vi "xyz-dh_express.vi"(0 "Image":dbl[][](array[numeric]), 1 "FFT":T2, 2 "Sizes":T1, 5 "R":dbl, 9 "Threshold type":u16(ring) items=["Top fraction", "Top value"], 11 "Threshold":dbl=2.0, 12 "FFT allocated?":bool=TRUE, 13 "mid_rng":dbl) -> (4 "XYZ":dbl[](array[numeric]), 6 "G":dbl[][](graph), 8 "Gx":dbl[][](graph), 10 "Gy":dbl[][](graph), 14 "dR":dbl[](array[numeric]), 15 "Filtered G":dbl[][](graph))   [LabVIEW 2015]
doc: "Single vi for calculating XYZ position of the particle.\n\nINPUT\nImage - input image\nR - radius of the window (should be >0.5)\nThreshold type, - type of threshold to apply:\n \"Top fraction\" - sets threshold as max_intensity/Threshold, e.g., for a Threshold=2 the threshold will be set to half the maximum pixel value \n \"Top value\" - sets the threshold to Threshold\nThreshold - threshold value\nFFT allocated? - must be set to true (default) if FFT and Sizes are connected. If set to False, FFT and Sizes inputs are ignored\nFFT, Sizes - Fourier transforms and sizes obtained from Local gradient preallocation\nPositive angle - angle in degrees that defines orientation of the image of the particle which corresponds to positive z-value\n\nOUTPUT\nXYZ - x,y position of the particle in pixels (for original image), z-value\nFiltered G - filtered local gradient magnitude image\nG,Gx,Gy - magnitude, horizontal and vertical local gradients correspondingly.\ndR - distance from the center to each line (1D vector)\n\nAuthor: Anatolii Kashchuk"
panel:
  in  "Weights type":u16(ring)=1 items=["None", "G", "G^2"]
  # "Author: Anatolii Kashchuk"
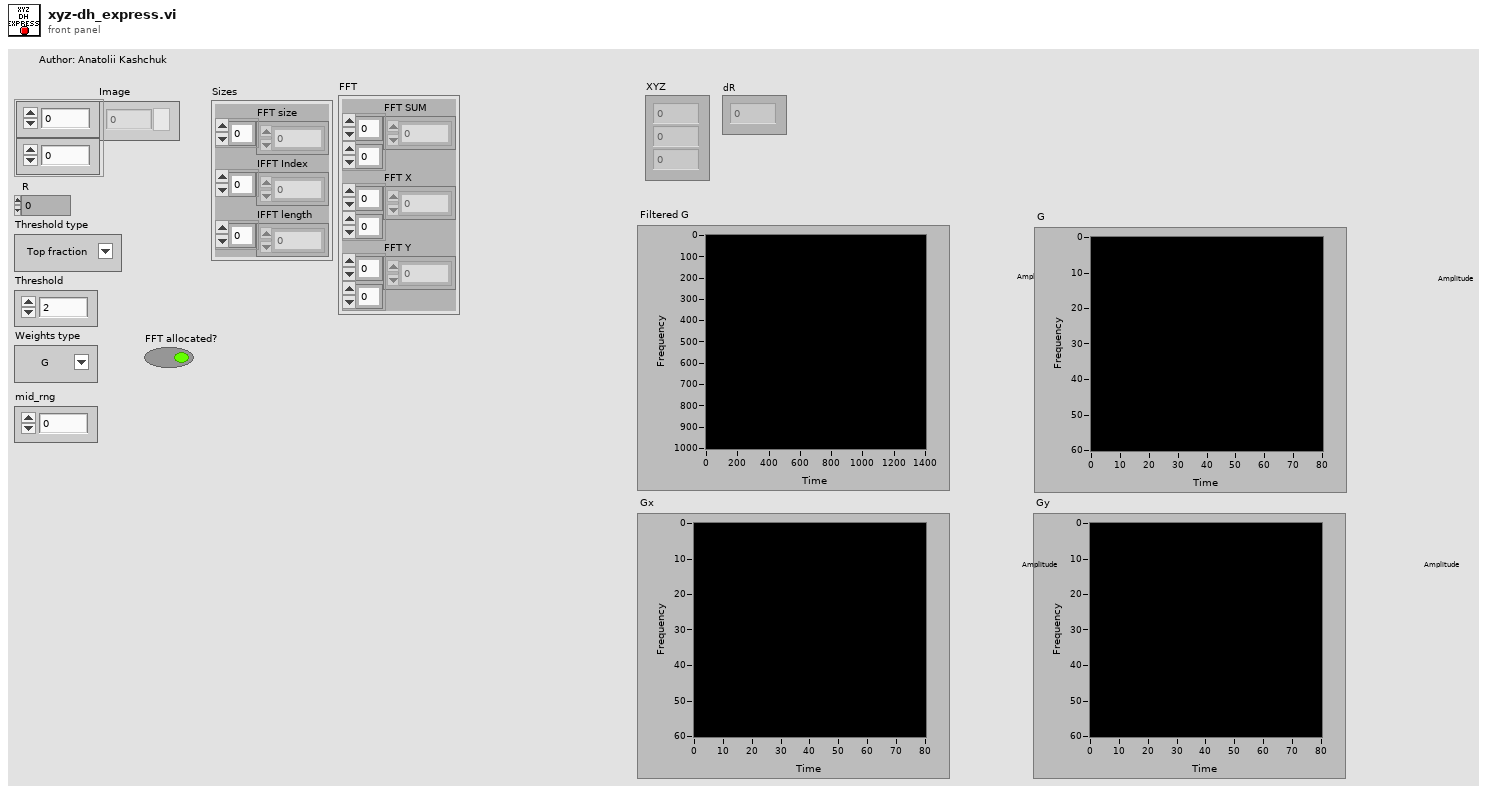
[diagram p1: front panel]
types:
  T1 = cluster{"FFT size":u32[], "IFFT Index":i32[], "IFFT length":u32[]}
  T2 = cluster{"FFT SUM":cdb[][], "FFT X":cdb[][], "FFT Y":cdb[][]}
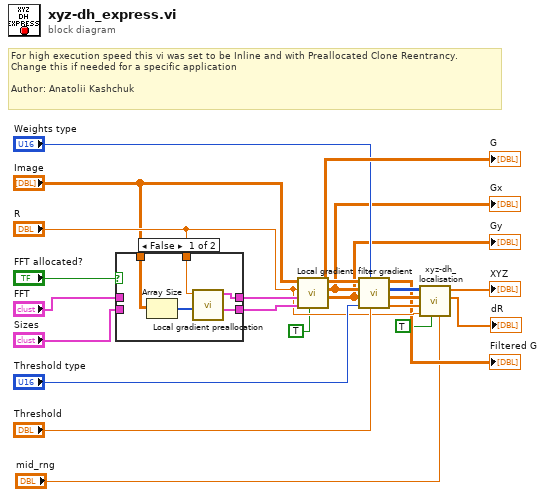
[diagram p0: block diagram]
diagram:
  # "For high execution speed this vi was set to be Inline and with Preallocated Clone Reentrancy. \nChange this if needed for a specific application\n\nAuthor: Anatolii Kashchuk"
  n1 = case shown="False" "FFT allocated?" {
    tunnel: [w27 w29] -> w19
    tunnel: [w26 w28] -> w18
    tunnel: "FFT" -> [_ w29]
    tunnel: "Sizes" -> [_ w28]
    tunnel: "R" -> [w25 _]
    tunnel: "Image" -> [w23 _]
    frame False {
      n2 = Array Size(array=w23) -> (size(s)=w24:i32[])
      n3 = call "Local gradient preallocation.vi"("Image size"=w24, "R"=w25) -> ("Sizes"=w26:T1, "FFT"=w27:T2)  [unwired: 8 in]
    }
    frame True {
    }
  }
  n4 = call "Local gradient.vi"("FFT allocated?"=TRUE, "Sizes"=w18, "FFT"=w19, "R"="R", "Image"="Image") -> ("Gy"=w10:dbl[][], "Gx"=w11:dbl[][], "G"=w22:dbl[][])  [unwired: 4 in]
  "Gy" <- w10
  "Gx" <- w11
  "G" <- w22
  n5 = call "filter gradient.vi"("Threshold"="Threshold", "Weights type"="Weights type", "Threshold type"="Threshold type", "Gy"=w10, "Gx"=w11, "G"=w22) -> ("Weights"=w12:dbl[], "gradients"=w13:dbl[][], "centers"=w14:i32[][], "Filtered G"=→"Filtered G":dbl[][])  [unwired: 2 out]
  n6 = call "xyz-dh_localisation.vi"("mid_rng"="mid_rng", "calculate z?"=TRUE, "R"="R", "weights"=w12, "B points"=w13, "A points"=w14) -> ("dR"=→"dR":dbl[], "XYZ"=→"XYZ":dbl[])  [unwired: 4 in]
